vi "Write Angle To Turn.vi"(8 "error in (no error)":errorcluster, 10 "Angle To Turn":dbl, 11 "TurnInstruction in":refnum<class "TurnInstruction.lvclass">) -> (0 "error out":errorcluster, 3 "TurnInstruction out":refnum<class "TurnInstruction.lvclass">)   [LabVIEW 2015, in "TurnInstruction.lvclass"]
uses:
  TurnInstruction.lvclass
  TurnInstruction.lvclass/TurnInstruction.ctl
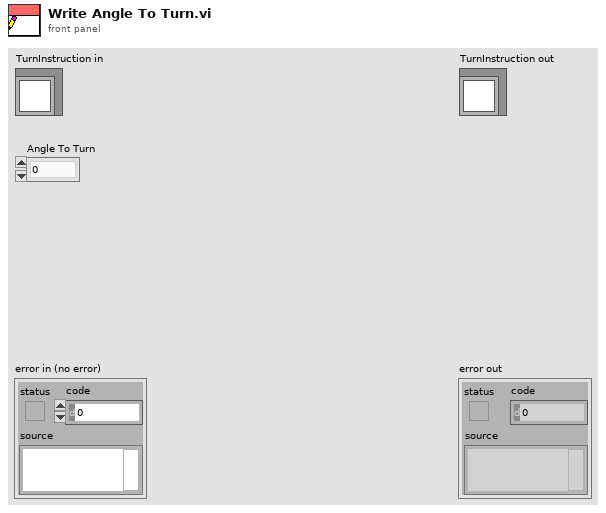
[diagram p1: front panel]
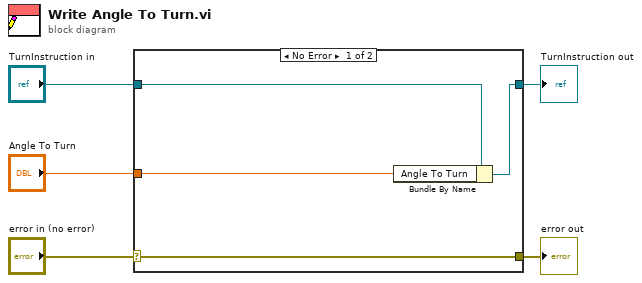
[diagram p0: block diagram]
diagram:
  n1 = case shown="No Error" "error in (no error)" {
    selector: "error in (no error)" -> [w9 w10]
    tunnel: [w9 w10] -> w4
    tunnel: [w7 w11] -> w2
    tunnel: "TurnInstruction in" -> [w8 w11]
    tunnel: "Angle To Turn" -> [w6 _]
    frame No Error {
      n2 = Bundle By Name(cluster=w8, "Angle To Turn"=w6) -> (w7:refnum<class "TurnInstruction.lvclass">)
    }
    frame Error {
    }
  }
  "error out" <- w4
  "TurnInstruction out" <- w2
